vi "Transform3d_Inverse.vi"(11 "inTransform3d":T1={"TRANSLATION3D"={"X"=0.0, "Y"=0.0, "Z"=0.0}, "ROTATION3D"={"Q_quaternion"={"R"=1.0, "V"=[0.0, 0.0, 0.0]}}, "XF"=FALSE} {"TRANSLATION3D"."Z" format="%14.3f"; "TRANSLATION3D"."Y" format="%14.3f"; "TRANSLATION3D"."X" format="%14.3f"}) -> (3 "outTransform3d":T1={"TRANSLATION3D"={"X"=0.0, "Y"=0.0, "Z"=0.0}, "ROTATION3D"={"Q_quaternion"={"R"=1.0, "V"=[0.0, 0.0, 0.0]}}, "XF"=FALSE} {"TRANSLATION3D"."Z" format="%14.3f"; "TRANSLATION3D"."Y" format="%14.3f"; "TRANSLATION3D"."X" format="%14.3f"})   [LabVIEW 2019, in "Trajectory_Library.lvlib"]
doc: "Invert the transformation3d. This is useful for undoing a transformation.\n\nParameters:\n - IN TRANSFORM3D -- This TRANSFORM3d data structure\n\nResults:\n - OUT TRANSFORM3D -- The inverted transformation."
uses:
  Trajectory_Library.lvlib
  TypeDef/TRANSLATION3D.ctl
  TypeDef/QUATERNION.ctl
  TypeDef/ROTATION3D.ctl
  TypeDef/TRANSFORM3D.ctl
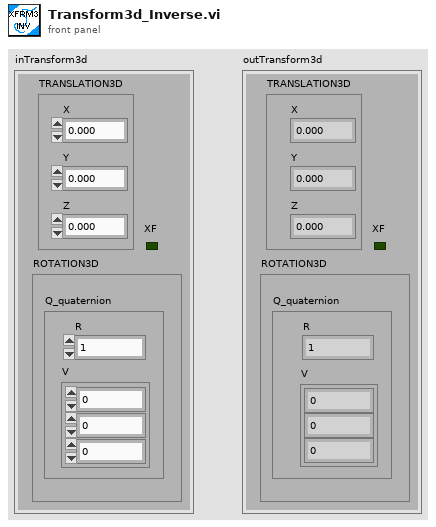
[diagram p1: front panel]
types:
  T1 = typedef "Trajectory_Library.lvlib/TRANSFORM3D.ctl" = cluster{"TRANSLATION3D":T2, "ROTATION3D":T3, "XF":bool}
  T2 = typedef "Trajectory_Library.lvlib/TRANSLATION3D.ctl" = cluster{"X":dbl, "Y":dbl, "Z":dbl}
  T3 = typedef "Trajectory_Library.lvlib/ROTATION3D.ctl" = cluster{"Q_quaternion":T4}
  T4 = typedef "Trajectory_Library.lvlib/QUATERNION.ctl" = cluster{"R":dbl, "V":dbl[]}
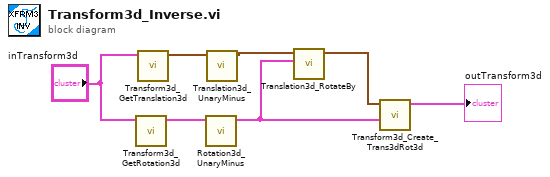
[diagram p0: block diagram]
diagram:
  n1 = call "Transform3d_GetRotation3d.vi"("in Transform3d"="inTransform3d") -> ("Rotation3d"=w3:T3)  [unwired: 10 in]
  n2 = call "Transform3d_GetTranslation3d.vi"("in Transform3d"="inTransform3d") -> ("Translation3d"=w5:T2)  [unwired: 10 in]
  n3 = call "Rotation3d_UnaryMinus.vi"("in Rotation3d"=w3) -> ("out Rotation3d"=w1:T3)  [unwired: 10 in]
  n4 = call "Translation3d_UnaryMinus.vi"("In Translation3d"=w5) -> ("Out Translation3d"=w2:T2)  [unwired: 10 in]
  n5 = call "Translation3d_RotateBy.vi"("other Rot3d"=w1, "in Translation3D"=w2) -> ("out Translation3d"=w6:T2)  [unwired: 9 in]
  n6 = call "Transform3d_Create_Trans3dRot3d.vi"("Rotation3d"=w1, "Translation3d"=w6) -> ("Transform3d"=→"outTransform3d":T1)  [unwired: 9 in]
